vi "mt_saveundload.vi"() -> ()   [LabVIEW 2022 SP3]
uses:
  <vilib>/Utility/file.llb/Read Delimited Spreadsheet (string).vi
  <vilib>/Utility/file.llb/Write Delimited Spreadsheet (string).vi
panel:
  out "Load":string[][](array[string])
  out "Process":string[][](array[string])
  in  "停止":bool
  in  "确定按钮":bool
  in  "布尔":bool
  in  "数值":dbl
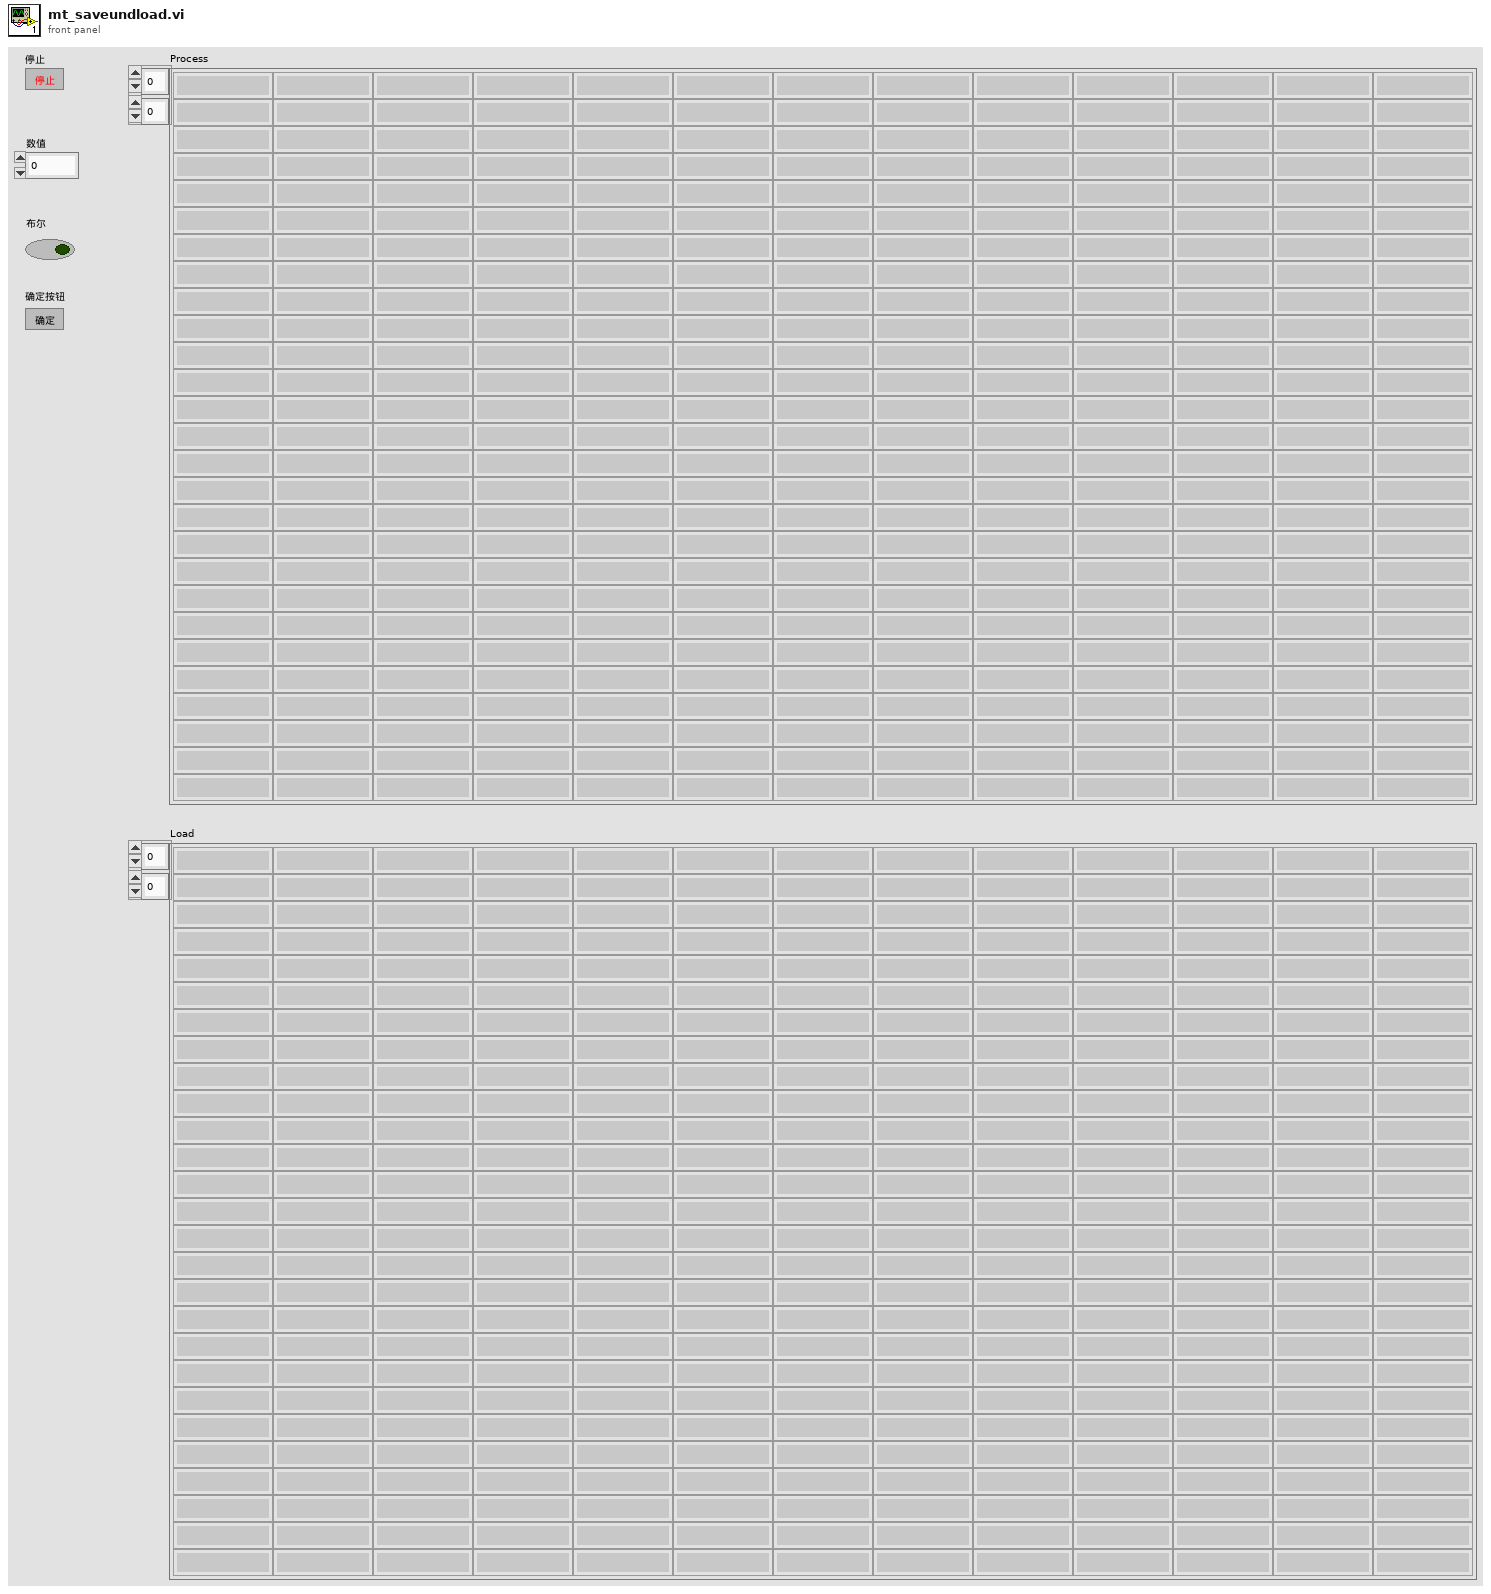
[diagram p1: front panel]
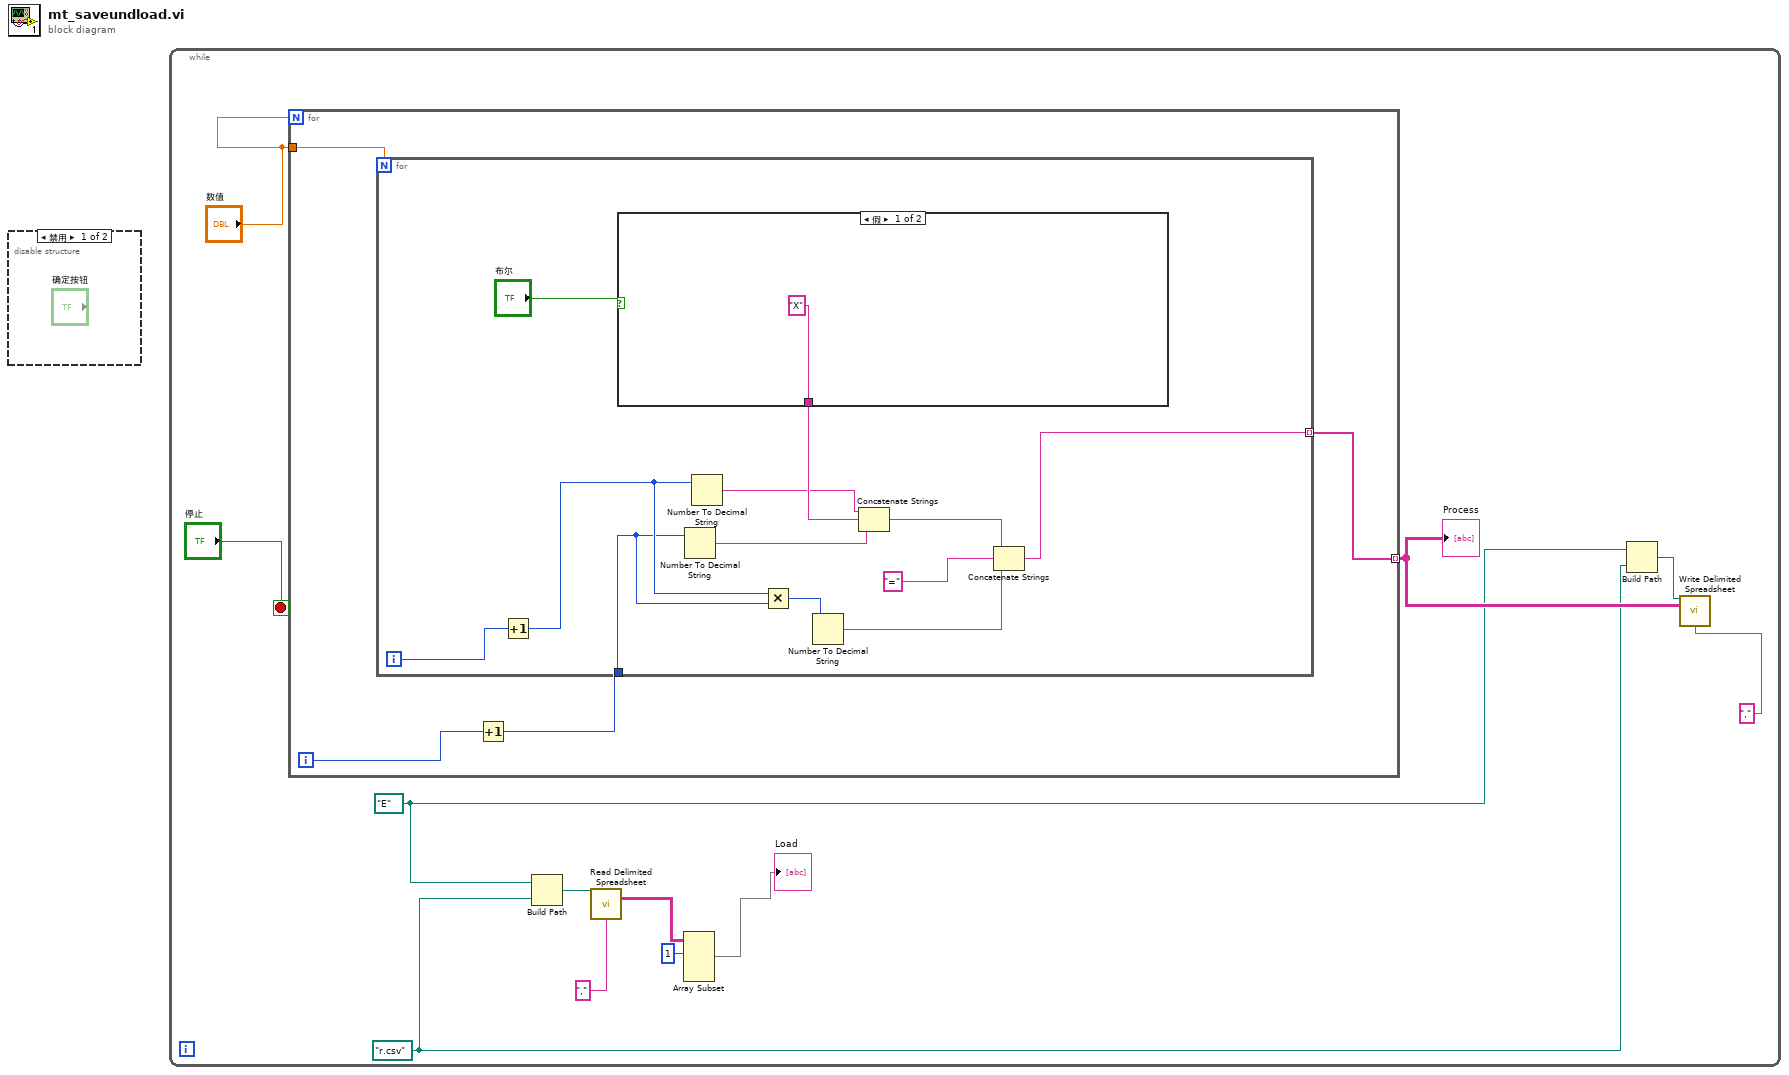
[diagram p0: block diagram]
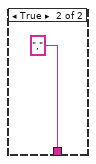
[diagram p3: hidden frame]
diagram:
  n1 = disable-structure shown="禁用" {
    frame Disabled {
    }
    frame Enabled {
    }
  }
  n2 = while {
    stop <- "停止" stop-if-true
    w2 = path "r.csv" ("名称或相对路径")
    w1 = path "E:/" ("基路径")
    n3 = for {
      N: "数值" -> [_]
      tunnel: "数值" -> [w16]
      tunnel: [w13] -> w10 mode=indexing
      i -> [w15]
      n4 = Increment(x=w15) -> (x+1=w14:i32)
      n5 = for {
        N: w16 -> [_]
        tunnel: w14 -> [w25]
        tunnel: [w17] -> w13 mode=indexing
        i -> [w27]
        n6 = Increment(x=w27) -> (x+1=w26:i32)
        n7 = case shown="假" "布尔" {
          tunnel: ["X" ","] -> w24
          frame False {
          }
          frame True {
          }
        }
        n8 = Number To Decimal String(number=w25) -> (decimal integer string=w22:string)  [unwired: 1 in]
        n9 = Number To Decimal String(number=w26) -> (decimal integer string=w23:string)  [unwired: 1 in]
        n10 = Multiply(x=w26, y=w25) -> (x*y=w19:i32)
        n11 = Number To Decimal String(number=w19) -> (decimal integer string=w18:string)  [unwired: 1 in]
        n12 = Concatenate Strings(w23, w24, w22) -> (w20:string)
        n13 = Concatenate Strings(w20, "=" ("字符串"), w18) -> (w17:string)
      }
    }
    "Process" <- w10
    n14 = Build Path(base path=w1, name or relative path=w2) -> (appended path=w5:path)
    n15 = call-poly <vilib>:"Read Delimited Spreadsheet.vi"("file path (dialog if empty)"=w5, "delimiter (\\t)"="," ("delimiter (\\t)")) -> ("all rows"=w6:string[][])  [unwired: 8 in, 5 out]
    n16 = Array Subset(array=w6, index (row)=1 ("索引")) -> (→"Load":string[][])  [unwired: 3 in]
    n17 = Build Path(base path=w1, name or relative path=w2) -> (appended path=w9:path)
    n18 = call-poly <vilib>:"Write Delimited Spreadsheet.vi"("file path (dialog if empty)"=w9, "2D data"=w10, "delimiter (\\t)"="," ("delimiter (\\t)")) -> ()  [unwired: 11 in, 2 out]
  }
